vi "Main.vi"() -> ()   [LabVIEW 2018]
uses:
  controls/Settings.ctl
  controls/LR Mode.ctl
  controls/Main Cluster.ctl
  classes/BKP-891 LCR Meter_class/BKP-891 LCR Meter.lvclass
  classes/BKP-911x Power Supply_class/BKP-911x Power Supply.lvclass
  classes/NI-DAQmx_class/NI-DAQmx.lvclass
  classes/Reporter_class/Reporter.lvclass
  classes/Tester_class/Tester.lvclass
  controls/IO Signal List.ctl
panel:
  in  "Tab Control":T1(tab)
  in  "UVW Mode":enum16{"UV", "UW", "VW"}(ring)
  in  "Signal Level (0:0.5 Vrms)":u8(ring) items=["0.5Vrms", "1Vrms"]
  in  "Signal Frequency (1000 Hz)":dbl=1000.0 format="%#_4g"
  in  "LR Mode":T2
  in  "Output Enabled":bool
  in  "Current Limit (A)":dbl
  in  "Voltage Setpoint (V)":dbl
  in  "Save Settings":bool
  in  "Settings":T3={"LCR VISA Resource"="", "PSU VISA Resource"="", "AI Task"="AI_Task", "AO Task"="AO_Task", "DO Task"="DO_Task", "Report Directory"=path ""}
  in  "exit":bool
  # "Gates EWP EOL Tester"
  # "BK Precision 891 - LCR Meter"
  # "NI cDAQ - Data Acquisition"
  # "BK Precision 9115 - Power Supply"
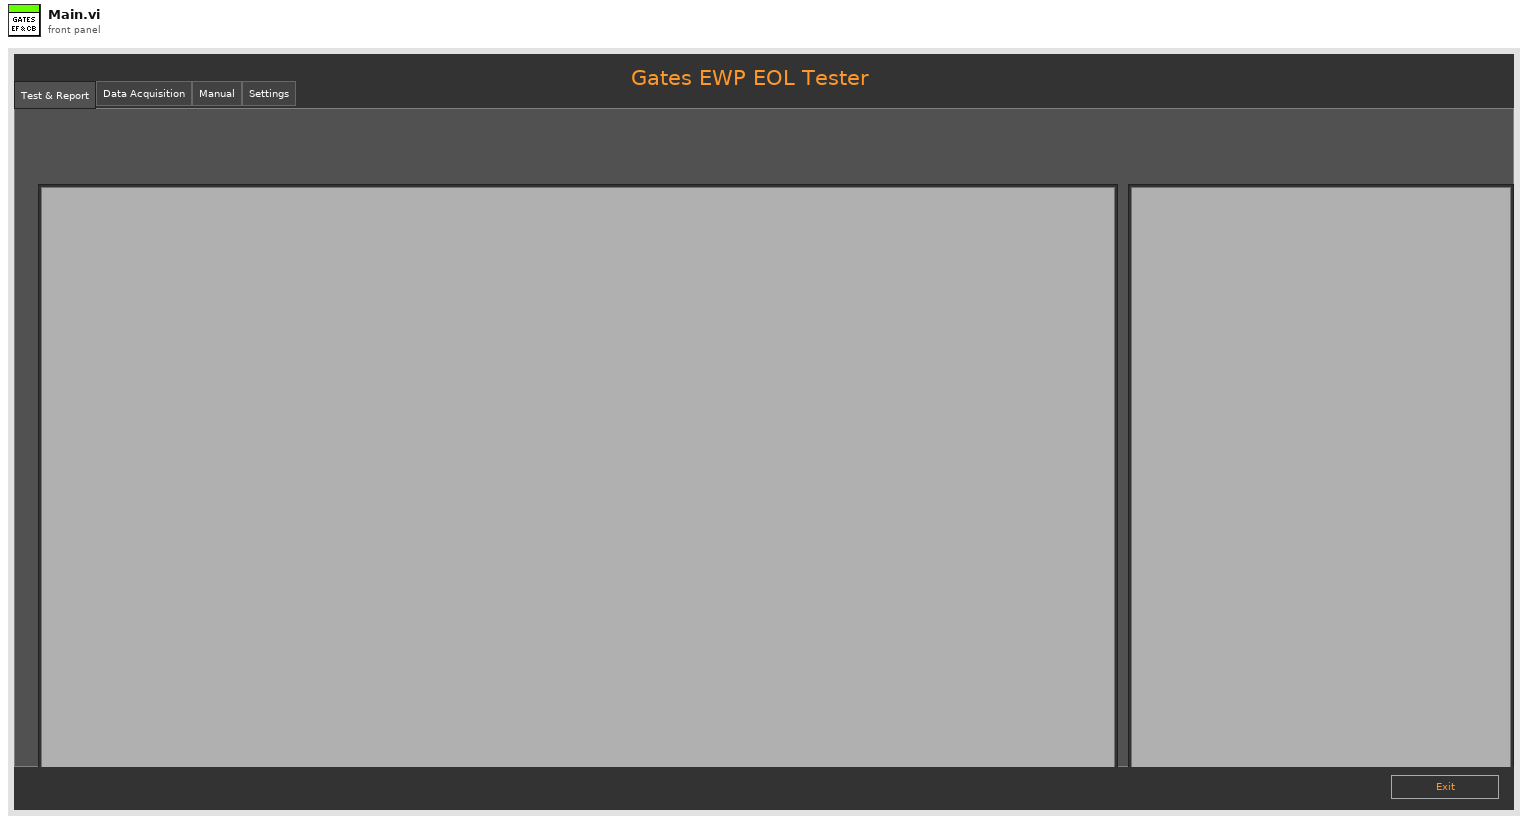
[diagram p1: front panel]
types:
  T1 = enum32{"Test & Report", "Data Acquisition", "Manual", "Settings"}
  T2 = typedef "LR Mode.ctl" = enum16{"R - Resistance", "L - Inductance"}
  T3 = typedef "Settings.ctl" = cluster{"LCR VISA Resource":refnum<visa-resource-name>, "PSU VISA Resource":refnum<visa-resource-name>, "AI Task":refnum<k21>, "AO Task":refnum<k21>, "DO Task":refnum<k21>, "Report Directory":path}
  T4 = typedef "Main Cluster.ctl" = cluster{"LCR":refnum<class "BKP-891 LCR Meter.lvclass">, "PSU":refnum<class "BKP-911x Power Supply.lvclass">, "NI-DAQmx":refnum<class "NI-DAQmx.lvclass">, "Reporter":refnum<class "Reporter.lvclass">, "Tester":refnum<class "Tester.lvclass">, "Settings":T3}
  T5 = typedef "IO Signal List.ctl" = enum16{"Timestamp", "PSU_FB_U_VDC", "PSU_FB_I_AMP", "PSU_FB_W_WATT", "PSU_CMD_U_VDC", "PSU_CMD_I_AMP", "PSU_CMD_OUTPUT", "LCR_PRIMARY", "LCR_SECONDARY", "UV_R_mOhm", "UW_R_mOhm", "VW_R_mOhm", "UV_L_µH", "UW_L_µH", "VW_L_µH", "U_U_VDC", "V_U_VDC", "W_U_VDC", "U_I_AMP", "V_I_AMP", "W_I_AMP", "PWM_CMD_DC_%", "PWM_CMD_VDC", "PWM_CMD_Hz", "PWM_FB_DC_%", "PWM_FB_VDC", "PWM_FB_Hz", "DO_RELAY_U_LCR_A", "DO_RELAY_V_LCR_A", "DO_RELAY_V_LCR_B", "DO_RELAY_W_LCR_B", "DIFF_UV_UW_L_µH", "DIFF_UV_VW_L_µH", "DIFF_UW_VW_L_µH", "DIFF_UV_UW_R_mOhm", "DIFF_UV_VW_R_mOhm", "DIFF_UW_VW_R_mOhm", "DIFF_UV_U_VDC", "DIFF_UW_U_VDC", "DIFF_VW_U_VDC"}
  T6 = enum32{"invalid app kind", "Development System", "Run Time System", "Student Edition", "Embedded LabVIEW", "Evaluation", "Custom"}
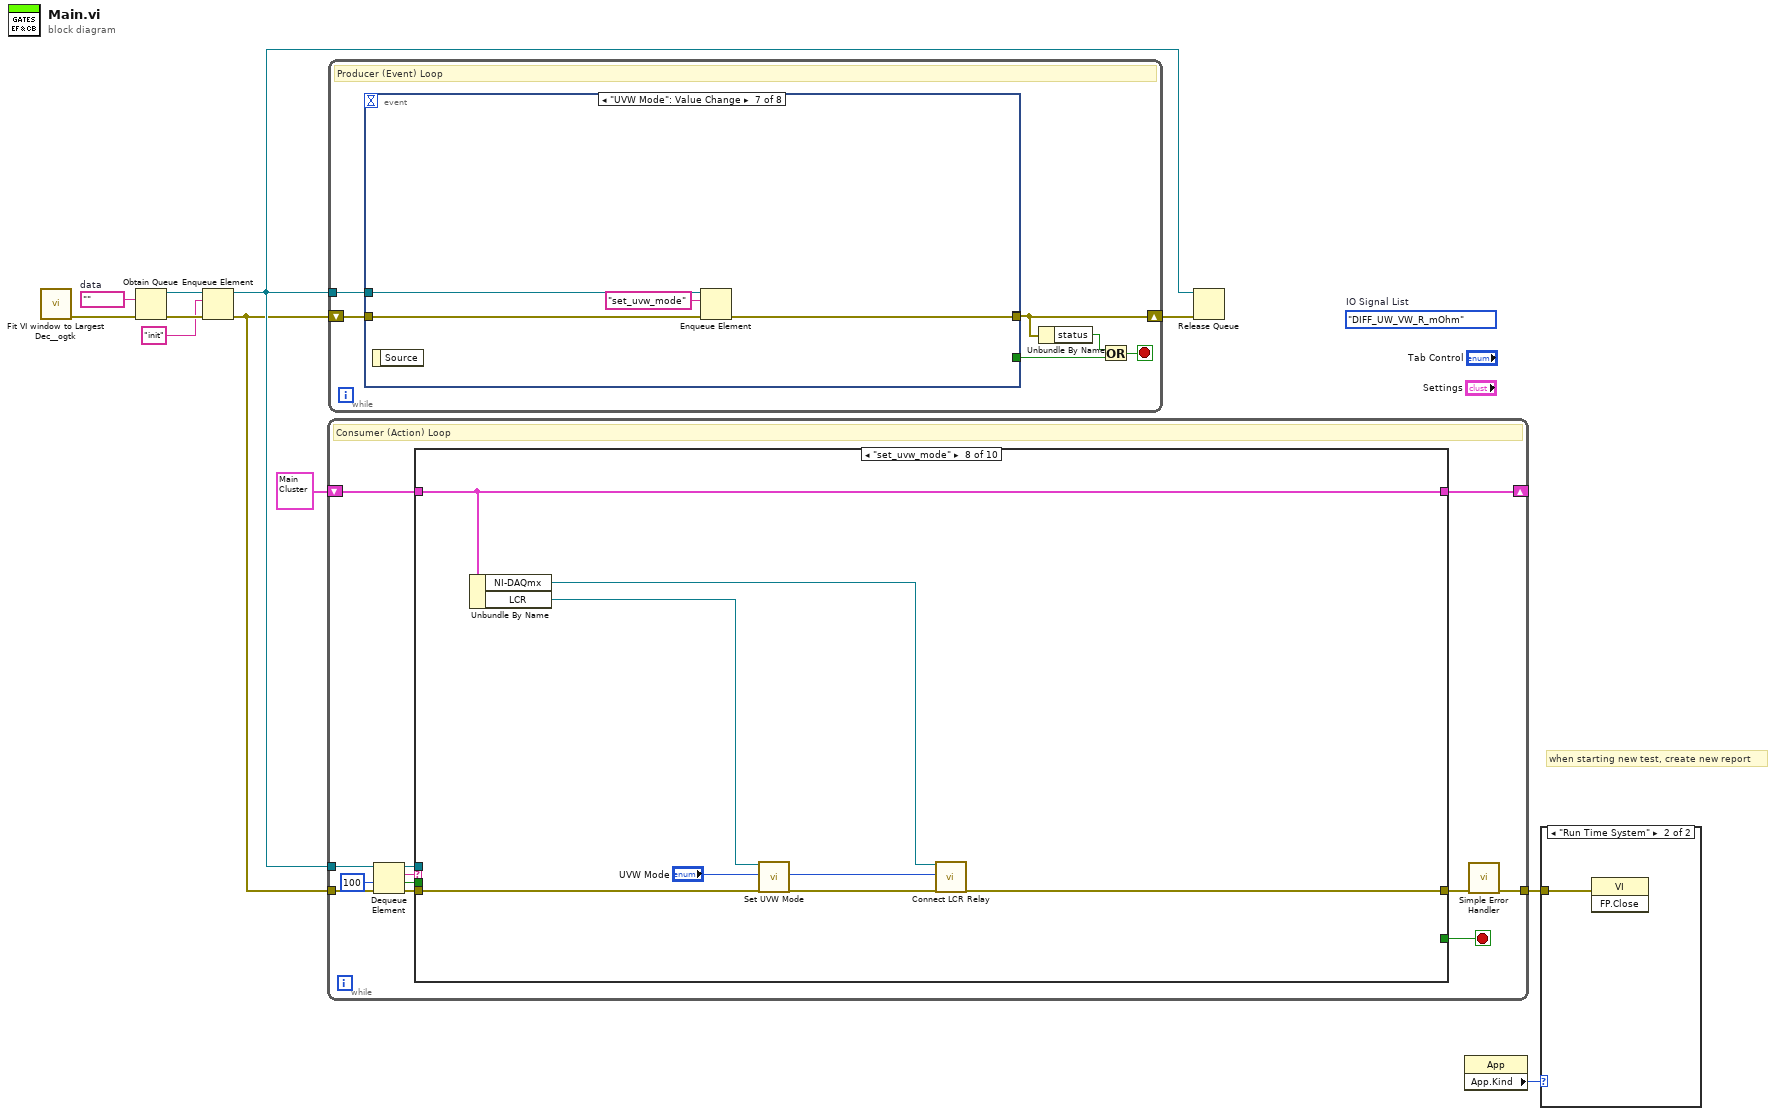
[diagram p0: block diagram]
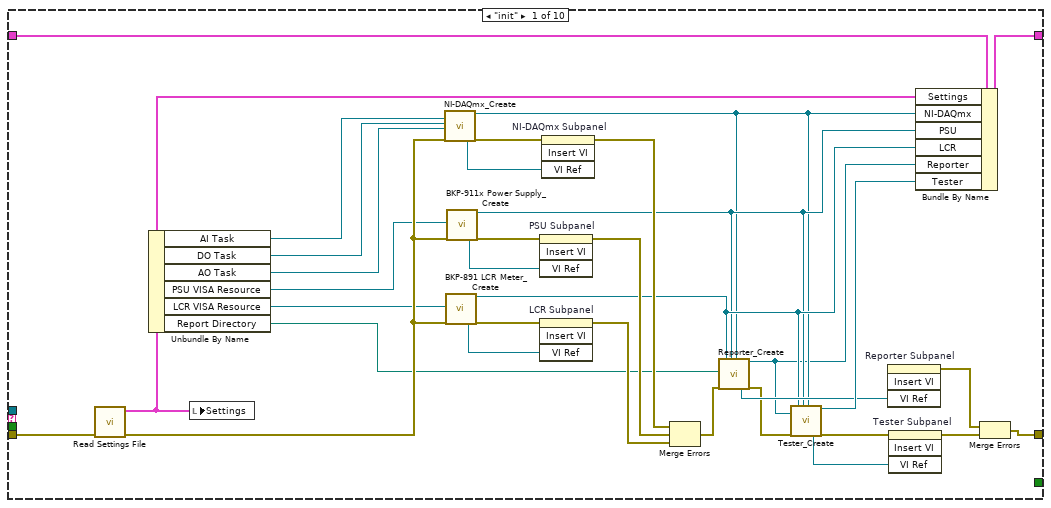
[diagram p3: hidden frame]
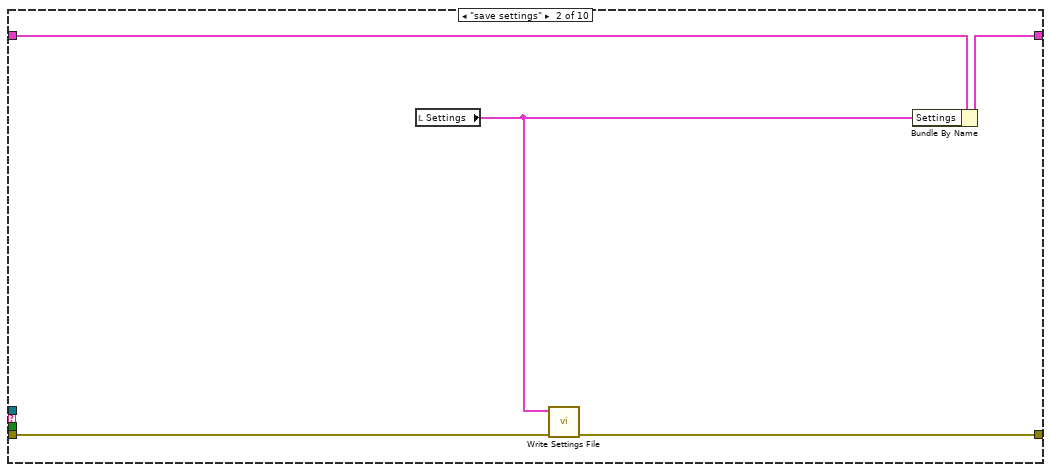
[diagram p4: hidden frame]
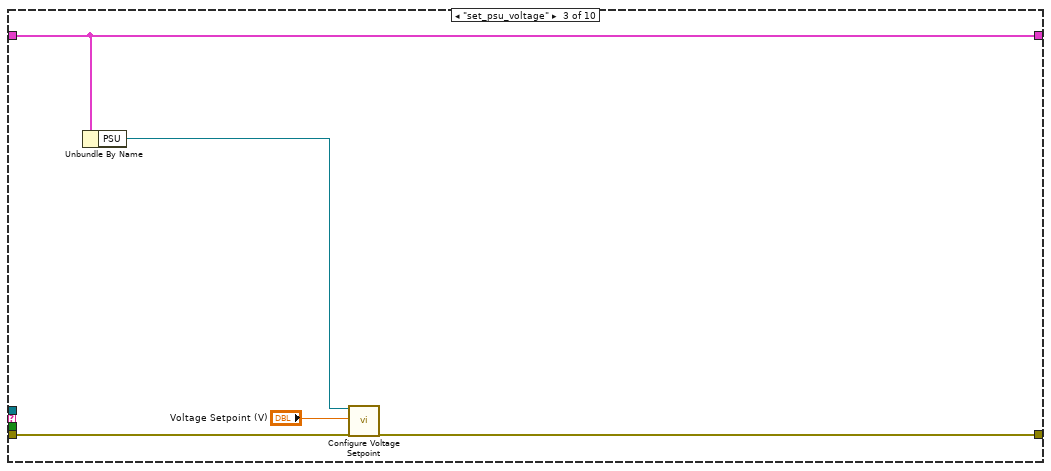
[diagram p5: hidden frame]
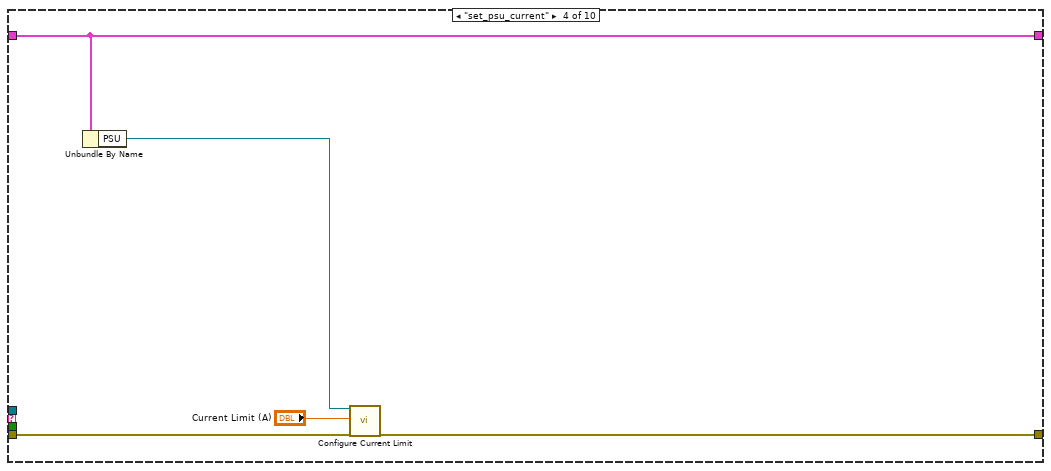
[diagram p6: hidden frame]
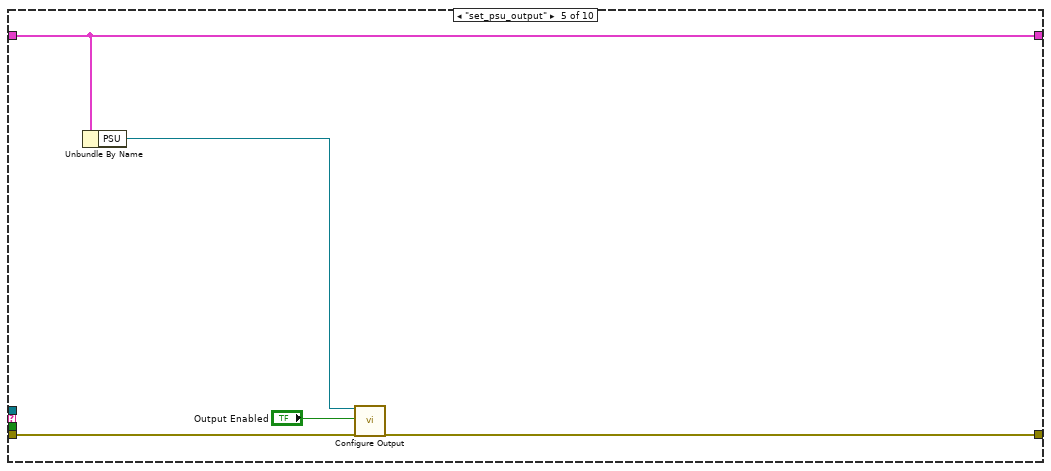
[diagram p7: hidden frame]
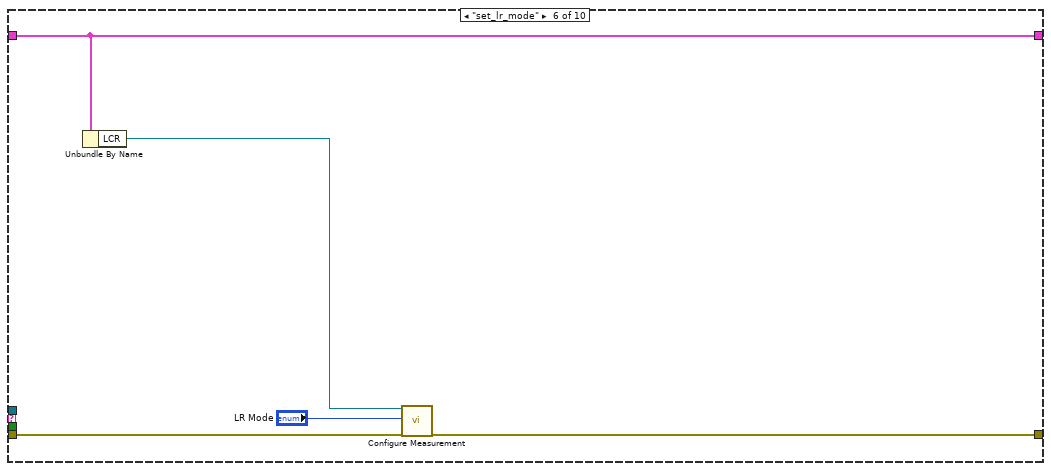
[diagram p8: hidden frame]
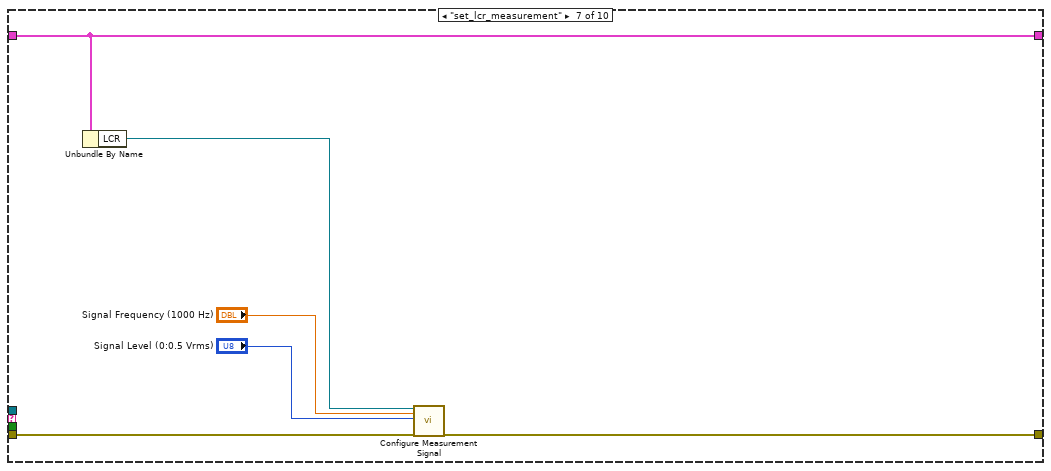
[diagram p9: hidden frame]
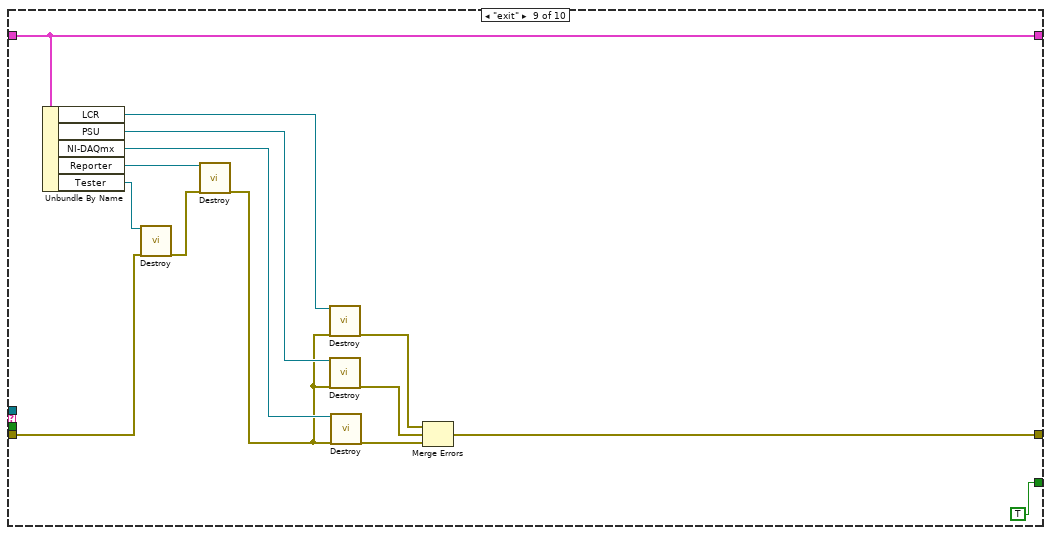
[diagram p10: hidden frame]
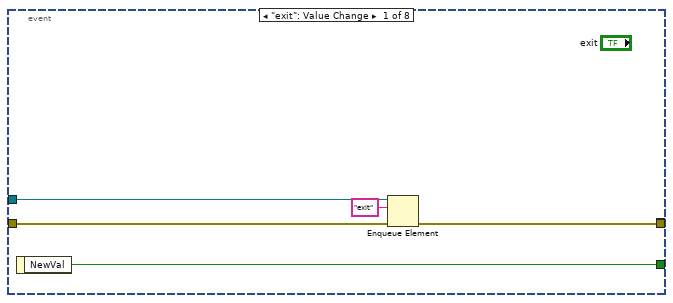
[diagram p12: hidden frame]
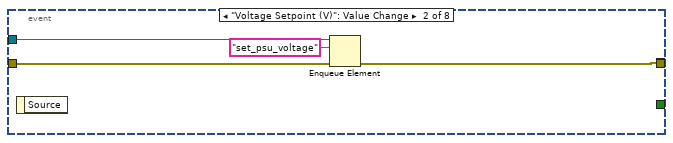
[diagram p13: hidden frame]
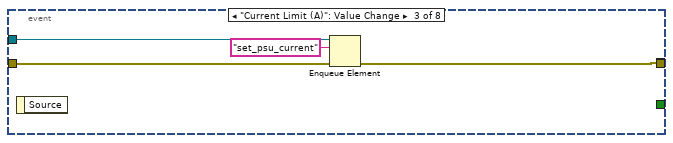
[diagram p14: hidden frame]
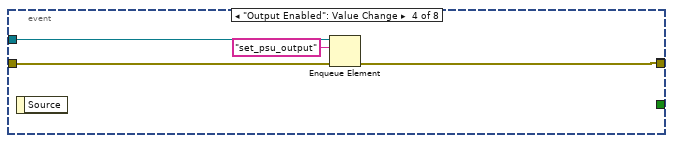
[diagram p15: hidden frame]
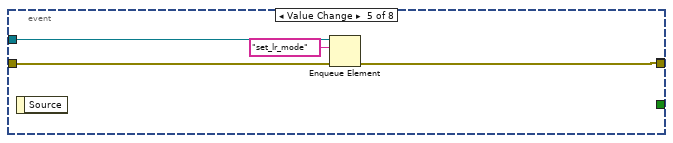
[diagram p16: hidden frame]
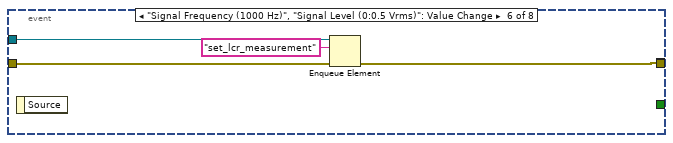
[diagram p17: hidden frame]
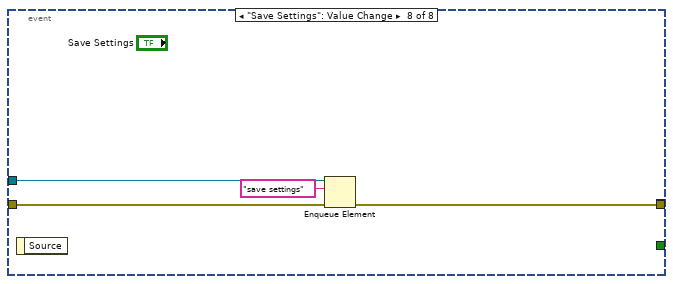
[diagram p18: hidden frame]
diagram:
  (unwired) IO_Signal_List."DIFF_UW_VW_R_mOhm"  # IO Signal List
  w10 = ""  # data
  # "when starting new test, create new report"
  n1 = call <userlib>:"Fit VI window to Largest Dec__ogtk.vi"() -> ("error out"=w9:errorcluster)  [unwired: 6 in, 1 out]
  n2 = Obtain Queue(element data type=w10, error in (no error)=w9) -> (queue out=w7:refnum<queue>, error out=w8:errorcluster)  [unwired: 3 in, 1 out]
  n3 = Enqueue Element(queue=w7, element="init", error in (no error)=w8) -> (queue out=w6:refnum<queue>, error out=w5:errorcluster)  [unwired: 1 in, 1 out]
  n4 = while {
    tunnel: w6 -> [w23]
    tunnel: w5 -> [w20]
    shift-right: [w17] -> _
    shift-left: T4 {"LCR"=refnum, "PSU"=refnum, "NI-DAQmx"=refnum, "Reporter"=refnum, "Tester"=refnum, "Settings"={"LCR VISA Resource"="", "PSU VISA Resource"="", "AI Task"="AI_Task", "AO Task"="AO_Task", "DO Task"="DO_Task", "Report Directory"=path ""}} -> [w18]
    tunnel: [w15] -> w1
    stop <- w22 stop-if-true
    # "Consumer (Action) Loop"
    n5 = Dequeue Element(queue=w23, timeout in ms (-1)=100, error in (no error)=w20) -> (queue out=w12:refnum<queue>, element=w21:string, timed out?=w13:bool, error out=w19:errorcluster)
    n6 = case shown="\"set_uvw_mode\"" w21 {
      tunnel: [_ _ _ _ _ _ _ _ TRUE _] -> w22
      tunnel: w19 -> [w43 w59 w65 w70 w75 w80 w85 w92 w105 w109]
      tunnel: w18 -> [w46 w61 w66 w71 w76 w81 w87 w94 w108 w110]
      tunnel: [w45 w60 w66 w71 w76 w81 w87 w94 w108 w110] -> w17
      tunnel: [w33 w57 w62 w69 w74 w79 w84 w88 w97 w109] -> w16
      tunnel: w13 -> [_ _ _ _ _ _ _ _ _ _]
      tunnel: w12 -> [_ _ _ _ _ _ _ _ _ _]
      frame "init" {
        n7 = call "Read Settings File.vi"("error in (no error)"=w43) -> ("error out"=w42:errorcluster, "Settings"=w25:T3)  [unwired: 9 in]
        n8 = Unbundle By Name(w25) -> ("AI Task"=w37:refnum<k21>, "DO Task"=w38:refnum<k21>, "AO Task"=w39:refnum<k21>, "PSU VISA Resource"=w40:refnum<visa-resource-name>, "LCR VISA Resource"=w41:refnum<visa-resource-name>, "Report Directory"=w24:path)
        n9 = local write "Settings"(w25) -> ()
        n10 = call "NI-DAQmx_Create.vi"("AI Task"=w37, "DO Task"=w38, "AO Task"=w39, "error in (no error)"=w42) -> ("ProcessViRef"=w53:refnum<vi>, "reference out"=w29:refnum<class "NI-DAQmx.lvclass">, "error out"=w54:errorcluster)  [unwired: 13 in]
        n11 = call "BKP-891 LCR Meter_Create.vi"("VISA resource name"=w41, "error in (no error)"=w42) -> ("ProcessViRef"=w55:refnum<vi>, "reference out"=w31:refnum<class "BKP-891 LCR Meter.lvclass">, "error out"=w56:errorcluster)  [unwired: 15 in]
        n12 = call "BKP-911x Power Supply_Create.vi"("VISA resource name"=w40, "error in (no error)"=w42) -> ("ProcessViRef"=w52:refnum<vi>, "reference out"=w30:refnum<class "BKP-911x Power Supply.lvclass">, "error out"=w51:errorcluster)  [unwired: 15 in]
        n13 = invoke on="PSU Subpanel" class="SubPnl" method="Insert VI"(error in=w51, "VI Ref"=w52) -> (error out=w50:errorcluster)  [unwired: 2 in, 3 out]
        n14 = invoke on="LCR Subpanel" class="SubPnl" method="Insert VI"(error in=w56, "VI Ref"=w55) -> (error out=w36:errorcluster)  [unwired: 2 in, 3 out]
        n15 = invoke on="NI-DAQmx Subpanel" class="SubPnl" method="Insert VI"(error in=w54, "VI Ref"=w53) -> (error out=w49:errorcluster)  [unwired: 2 in, 3 out]
        n16 = Merge Errors(w49, w50, w36) -> (w27:errorcluster)
        n17 = call "Reporter_Create.vi"("Report Directory"=w24, "error in (no error)"=w27, "LCR"=w31, "PSU"=w30, "NI-DAQmx"=w29) -> ("ProcessViRef"=w32:refnum<vi>, "reference out"=w28:refnum<class "Reporter.lvclass">, "error out"=w26:errorcluster)  [unwired: 12 in]
        n18 = call "Tester_Create.vi"("Reporter"=w28, "error in (no error)"=w26, "LCR"=w31, "PSU"=w30, "NI-DAQmx"=w29) -> ("ProcessViRef"=w47:refnum<vi>, "reference out"=w44:refnum<class "Tester.lvclass">, "error out"=w48:errorcluster)  [unwired: 12 in]
        n19 = invoke on="Reporter Subpanel" class="SubPnl" method="Insert VI"("VI Ref"=w32) -> (error out=w34:errorcluster)  [unwired: 3 in, 3 out]
        n20 = invoke on="Tester Subpanel" class="SubPnl" method="Insert VI"(error in=w48, "VI Ref"=w47) -> (error out=w35:errorcluster)  [unwired: 2 in, 3 out]
        n21 = Bundle By Name(cluster=w46, "Settings"=w25, "NI-DAQmx"=w29, "PSU"=w30, "LCR"=w31, "Reporter"=w28, "Tester"=w44) -> (w45:T4)
        n22 = Merge Errors(w34, w35) -> (w33:errorcluster)
      }
      frame "save settings" {
        n23 = local read "Settings"() -> (w58:T3)
        n24 = call "Write Settings File.vi"("error in (no error)"=w59, "Settings"=w58) -> ("error out"=w57:errorcluster)  [unwired: 9 in]
        n25 = Bundle By Name(cluster=w61, "Settings"=w58) -> (w60:T4)
      }
      frame "set_psu_voltage" {
        n26 = Unbundle By Name(w66) -> ("PSU"=w64:refnum<class "BKP-911x Power Supply.lvclass">)
        n27 = call-dynamic "Configure Voltage Setpoint.vi"("reference in"=w64, "Voltage Setpoint (V)"="Voltage Setpoint (V)", "error in (no error)"=w65) -> ("error out"=w62:errorcluster)  [unwired: 15 in, 1 out]
      }
      frame "set_psu_current" {
        n28 = Unbundle By Name(w71) -> ("PSU"=w68:refnum<class "BKP-911x Power Supply.lvclass">)
        n29 = call-dynamic "Configure Current Limit.vi"("reference in"=w68, "Current Limit (0.0 A)"="Current Limit (A)", "error in (no error)"=w70) -> ("error out"=w69:errorcluster)  [unwired: 15 in, 1 out]
      }
      frame "set_psu_output" {
        n30 = Unbundle By Name(w76) -> ("PSU"=w73:refnum<class "BKP-911x Power Supply.lvclass">)
        n31 = call-dynamic "Configure Output.vi"("reference in"=w73, "Enable Output (T: Enable)"="Output Enabled", "error in (no error)"=w75) -> ("error out"=w74:errorcluster)  [unwired: 15 in, 1 out]
      }
      frame "set_lr_mode" {
        n32 = Unbundle By Name(w81) -> ("LCR"=w78:refnum<class "BKP-891 LCR Meter.lvclass">)
        n33 = call-dynamic "Configure Measurement.vi"("reference in"=w78, "LR Mode"="LR Mode", "error in (no error)"=w80) -> ("error out"=w79:errorcluster)  [unwired: 15 in, 1 out]
      }
      frame "set_lcr_measurement" {
        n34 = Unbundle By Name(w87) -> ("LCR"=w86:refnum<class "BKP-891 LCR Meter.lvclass">)
        n35 = call-dynamic "Configure Measurement Signal.vi"("reference in"=w86, "Signal Frequency (1000 Hz)"="Signal Frequency (1000 Hz)", "Signal Level (0:0.5 Vrms)"="Signal Level (0:0.5 Vrms)", "error in (no error)"=w85) -> ("error out"=w84:errorcluster)  [unwired: 14 in, 1 out]
      }
      frame "set_uvw_mode" {
        n36 = Unbundle By Name(w94) -> ("NI-DAQmx"=w90:refnum<class "NI-DAQmx.lvclass">, "LCR"=w93:refnum<class "BKP-891 LCR Meter.lvclass">)
        n37 = call-dynamic "Set UVW Mode.vi"("reference in"=w93, "UVW Mode"="UVW Mode", "error in (no error)"=w92) -> ("error out"=w91:errorcluster)  [unwired: 15 in, 1 out]
        n38 = call-dynamic "Connect LCR Relay.vi"("reference in"=w90, "Relay Mode"="UVW Mode", "error in (no error)"=w91) -> ("error out"=w88:errorcluster)  [unwired: 15 in, 1 out]
      }
      frame "exit" {
        n39 = Unbundle By Name(w108) -> ("LCR"=w102:refnum<class "BKP-891 LCR Meter.lvclass">, "PSU"=w103:refnum<class "BKP-911x Power Supply.lvclass">, "NI-DAQmx"=w104:refnum<class "NI-DAQmx.lvclass">, "Reporter"=w106:refnum<class "Reporter.lvclass">, "Tester"=w107:refnum<class "Tester.lvclass">)
        n40 = call-dynamic "Destroy.vi"("reference in"=w107, "error in (no error)"=w105) -> ("error out"=w96:errorcluster)  [unwired: 16 in, 1 out]
        n41 = call-dynamic "Destroy.vi"("reference in"=w106, "error in (no error)"=w96) -> ("error out"=w95:errorcluster)  [unwired: 16 in, 1 out]
        n42 = call-dynamic "Destroy.vi"("reference in"=w102, "error in (no error)"=w95) -> ("error out"=w101:errorcluster)  [unwired: 16 in, 1 out]
        n43 = call-dynamic "Destroy.vi"("reference in"=w103, "error in (no error)"=w95) -> ("error out"=w100:errorcluster)  [unwired: 16 in, 1 out]
        n44 = call-dynamic "Destroy.vi"("reference in"=w104, "error in (no error)"=w95) -> ("error out"=w99:errorcluster)  [unwired: 16 in, 1 out]
        n45 = Merge Errors(w101, w100, w99) -> (w97:errorcluster)
      }
      frame Default {
      }
    }
    n46 = call <vilib>:"Simple Error Handler.vi"("error in (no error)"=w16) -> ("error out"=w15:errorcluster)  [unwired: 4 in, 4 out]
  }
  n47 = while {
    shift-right: [w112] -> w11
    shift-left: w5 -> [w115]
    tunnel: w6 -> [w116]
    stop <- w113 stop-if-true
    # "Producer (Event) Loop"
    n48 = event shown="[6] \"UVW Mode\": Value Change" {
      selector: _ -> [_ _ _ _ _ _ _ _]
      dyn-events: _ -> [_ _ _ _ _ _ _ _]
      timeout: _ -> [_ _ _ _ _ _ _ _]
      tunnel: w116 -> [w119 w124 w128 w132 w136 w140 w143 w148]
      tunnel: w115 -> [w120 w125 w129 w133 w137 w141 w144 w149]
      tunnel: [w117 w122 w126 w130 w134 w138 _ w146] -> w112
      tunnel: [w121 _ _ _ _ _ _ _] -> w114
      tunnel: [_ _ _ _ _ _ w142 _] -> _
      event "exit": Value Change {
        n49 = event-data() -> ("NewVal"=w121:bool)  [unwired: 1 in]
        n50 = Enqueue Element(queue=w119, element="exit", error in (no error)=w120) -> (error out=w117:errorcluster)  [unwired: 1 in, 2 out]
      }
      event "Voltage Setpoint (V)": Value Change {
        n51 = event-data() -> ()  [unwired: 1 in, 1 out]
        n52 = Enqueue Element(queue=w124, element="set_psu_voltage", error in (no error)=w125) -> (error out=w122:errorcluster)  [unwired: 1 in, 2 out]
      }
      event "Current Limit (A)": Value Change {
        n53 = event-data() -> ()  [unwired: 1 in, 1 out]
        n54 = Enqueue Element(queue=w128, element="set_psu_current", error in (no error)=w129) -> (error out=w126:errorcluster)  [unwired: 1 in, 2 out]
      }
      event "Output Enabled": Value Change {
        n55 = event-data() -> ()  [unwired: 1 in, 1 out]
        n56 = Enqueue Element(queue=w132, element="set_psu_output", error in (no error)=w133) -> (error out=w130:errorcluster)  [unwired: 1 in, 2 out]
      }
      event Value Change {
        n57 = event-data() -> ()  [unwired: 1 in, 1 out]
        n58 = Enqueue Element(queue=w136, element="set_lr_mode", error in (no error)=w137) -> (error out=w134:errorcluster)  [unwired: 1 in, 2 out]
      }
      event "Signal Frequency (1000 Hz)", "Signal Level (0:0.5 Vrms)": Value Change {
        n59 = event-data() -> ()  [unwired: 1 in, 1 out]
        n60 = Enqueue Element(queue=w140, element="set_lcr_measurement", error in (no error)=w141) -> (error out=w138:errorcluster)  [unwired: 1 in, 2 out]
      }
      event "UVW Mode": Value Change {
        n61 = event-data() -> ()  [unwired: 1 in, 1 out]
        n62 = Enqueue Element(queue=w143, element="set_uvw_mode", error in (no error)=w144) -> (error out=w142:errorcluster)  [unwired: 1 in, 2 out]
      }
      event "Save Settings": Value Change {
        n63 = event-data() -> ()  [unwired: 1 in, 1 out]
        n64 = Enqueue Element(queue=w148, element="save settings", error in (no error)=w149) -> (error out=w146:errorcluster)  [unwired: 1 in, 2 out]
      }
    }
    n65 = Unbundle By Name(w112) -> ("status"=w111:bool)
    n66 = Or(x=w111, y=w114) -> (x .or. y?=w113:bool)
  }
  n67 = Release Queue(queue=w6, error in (no error)=w11) -> ()  [unwired: 1 in, 3 out]
  n68 = property class="App"() -> ("App.Kind"=w2:T6)  [unwired: 2 in, 2 out]
  n69 = case shown="\"Run Time System\"" w2 {
    tunnel: w1 -> [_ w150]
    frame Default {
    }
    frame "Run Time System" {
      n70 = invoke class="VI" method="FP.Close"(error in=w150) -> ()  [unwired: 2 in, 3 out]
    }
  }
